vi "WhileYShiftRegister.vi"() -> ()   [LabVIEW 2022 SP3]
panel:
  out "Waveform Chart":dbl(graph)
  in  "stop":bool
  out "Número aleatorio":dbl
  in  "Límite inferior":dbl
  in  "Límite superior":dbl
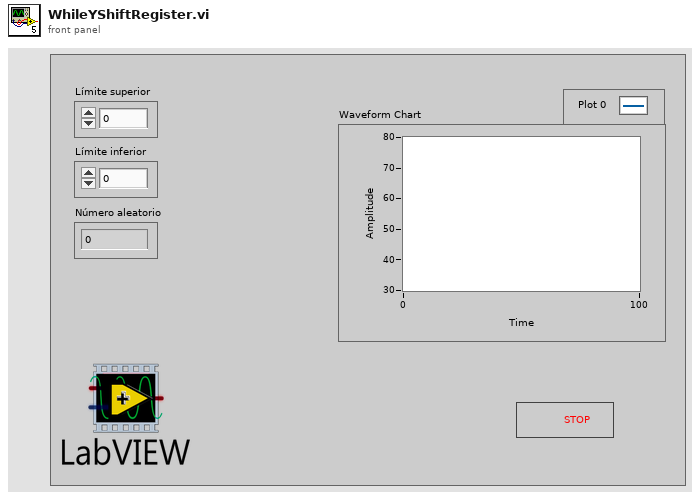
[diagram p1: front panel]
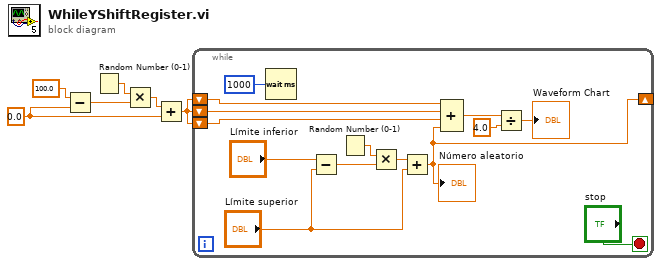
[diagram p0: block diagram]
diagram:
  w2 = 0.0 ("y")
  n1 = Subtract(x=100.0, y=w2) -> (x-y=w5:dbl)
  n2 = Random Number (0-1)() -> (number: 0 to 1=w4:dbl)
  n3 = Multiply(x=w4, y=w5) -> (x*y=w3:dbl)
  n4 = Add(x=w3, y=w2) -> (x+y=w1:dbl)
  n5 = while {
    shift-right: [w7] -> _
    shift-left: w1 -> [w13]
    shift-left: w1 -> [w11]
    shift-left: w1 -> [w12]
    stop <- "stop" stop-if-true
    n6 = Wait (ms)(milliseconds to wait=u32 1000) -> ()  [unwired: 1 out]
    n7 = Subtract(x="Límite inferior", y="Límite superior") -> (x-y=w18:dbl)
    n8 = Random Number (0-1)() -> (number: 0 to 1=w19:dbl)
    n9 = Multiply(x=w19, y=w18) -> (x*y=w17:dbl)
    n10 = Add(x=w17, y="Límite superior") -> (x+y=w7:dbl)
    "Número aleatorio" <- w7
    n11 = Compound Arithmetic op=ADD(w13, w12, w11, w7) -> (w10:dbl)
    n12 = Divide(x=w10, y=4.0) -> (x/y=→"Waveform Chart":dbl)
  }
